vi "Marker Draw and Commands Loop.vi"(4 "Cursor Options":T1={"font"={"Font Name"="Arial", "Size"=15, "Strikeout?"=FALSE, "Italic?"=FALSE, "Underline?"=FALSE, "Outline?"=FALSE, "Shadow?"=FALSE, "Bold?"=FALSE}, "size"=2, "Timestamp"=enum."at BOTTOM", "Vertical Line?"=TRUE, "Horizontal Line?"=TRUE, "alignment(left, top)"={"horizontal"=enum."left", "vertical"=enum."center"}, "TextFormat"=" %3$s\\n %2$.2f", "time format (%H:%M:%S)"="%I:%M:%S %p"} {"size" min=1 max=50}, 6 "Enable Cursors":bool, 9 "Markers":T2[](array[typedef]), 10 "XY Graph":refnum<vi>, 11 "Options":T4={"Color"=16723218, "pen"={"Width"=2, "Style"=enum."Solid"}, "font"={"Font Name"="Arial", "Size"=14, "Strikeout?"=FALSE, "Italic?"=FALSE, "Underline?"=FALSE, "Outline?"=FALSE, "Shadow?"=FALSE, "Bold?"=FALSE, "FontColor"=6908265}, "caption"="Click to set a point marker"}) -> ()   [LabVIEW 2020, in "Graph Extensions.lvlib"]
doc: "This draw loop is the command processor thread and redraw thread to handle the events from the UI. It can be started anywhere with a reference to the graph. Markers work only when the graph palette tool is in cursor mode, as it replaces that mode since Graph extensions have their own improved cursors/markers, that mode is not needed. \n\n<B>Options</B> can be changed by the user using the right click menu with the markers.\n<B>Markers</B> input can be used to initialize a known set of markers (eitehr loaded from disk or programmatically created)\n\n<B>Cursers Enabled</B> activates the other graph extension (cursors) when usual mouse move occurs."
uses:
  Graph Extensions.lvlib
  controls/MarkerOptions.ctl
  controls/MarkerInfo.ctl
  controls/markerType.ctl
  controls/CursorOptions.ctl
  controls/GraphExt-Cmds.ctl
  controls/commands.ctl
  <vilib>/Utility/miscctls.llb/LVPoint32TypeDef.ctl
  controls/cmd_options.ctl
  controls/Simple Global for Marker Options.vi
panel:
  in  "stop":bool
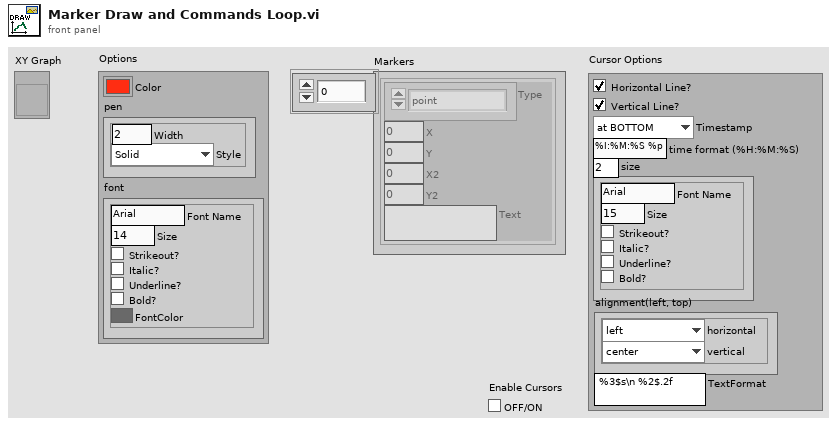
[diagram p1: front panel]
types:
  T1 = typedef "Graph Extensions.lvlib/CursorOptions.ctl" = cluster{"font":cluster{"Font Name":string, "Size":i16, "Strikeout?":bool, "Italic?":bool, "Underline?":bool, "Outline?":bool, "Shadow?":bool, "Bold?":bool}, "size":i16, "Timestamp":enum16{"at TOP", "at BOTTOM", "none"}, "Vertical Line?":bool, "Horizontal Line?":bool, "alignment(left, top)":cluster{"horizontal":enum16{"left", "center", "right"}, "vertical":enum16{"top", "center", "bottom"}}, "TextFormat":string, "time format (%H:%M:%S)":string}
  T2 = typedef "Graph Extensions.lvlib/MarkerInfo.ctl" = cluster{"Type":T3, "X":dbl, "Y":dbl, "X2":dbl, "Y2":dbl, "Text":string}
  T3 = typedef "Graph Extensions.lvlib/markerType.ctl" = enum16{"point", "arrow", "horiz", "vert", "vert range", "horiz range", "box"}
  T4 = typedef "Graph Extensions.lvlib/MarkerOptions.ctl" = cluster{"Color":u32, "pen":cluster{"Width":u16, "Style":enum32{"Solid", "Dash", "Dot", "DashDot", "DashDotDot"}}, "font":cluster{"Font Name":string, "Size":i16, "Strikeout?":bool, "Italic?":bool, "Underline?":bool, "Outline?":bool, "Shadow?":bool, "Bold?":bool, "FontColor":u32}, "caption":string}
  T5 = typedef "Graph Extensions.lvlib/commands.ctl" = enum16{"up", "options", "click", "move", "type", "redraw", "edited", "exit", "Mark"}
  T6 = typedef "LVPoint32TypeDef.ctl" = cluster{"Horizontal":i32, "Vertical":i32}
  T7 = cluster{"cmd":T5, "Type":T3, "Coords":T6, "Active Tool":i32, "mode":enum16{"drag", "none"}}
  T8 = typedef "Graph Extensions.lvlib/GraphExt-Cmds.ctl" = cluster{"cmd":T5, "Type":T3, "Coords":T6, "text":string}
  T9 = typedef "Graph Extensions.lvlib/cmd_options.ctl" = cluster{"Marker Color":u32, "Style":enum32{"Solid", "Dash", "Dot", "DashDot", "DashDotDot"}, "Width":u16, "Size":i16, "Color":u32}
  T10 = typedef "LVRectTypeDef.ctl" = cluster{"Left":i16, "Top":i16, "Right":i16, "Bottom":i16}
  T11 = enum32{"Solid", "Dash", "Dot", "DashDot", "DashDotDot"}
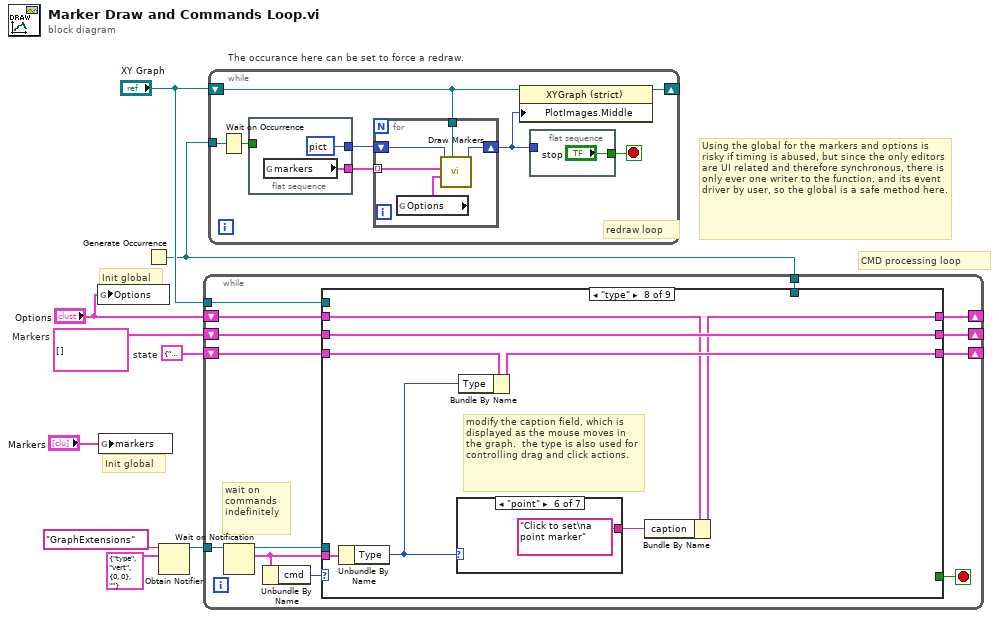
[diagram p0: block diagram]
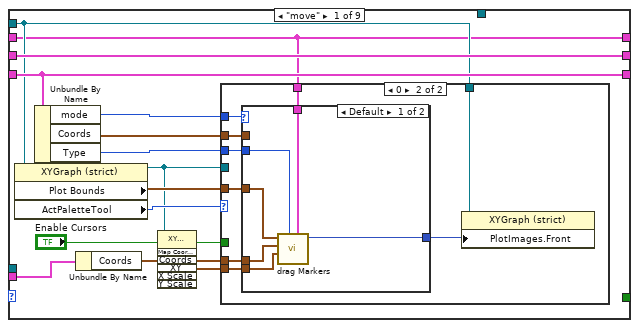
[diagram p2: hidden frame]
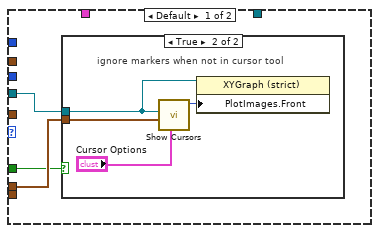
[diagram p3: hidden frame]
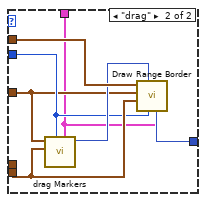
[diagram p5: hidden frame]
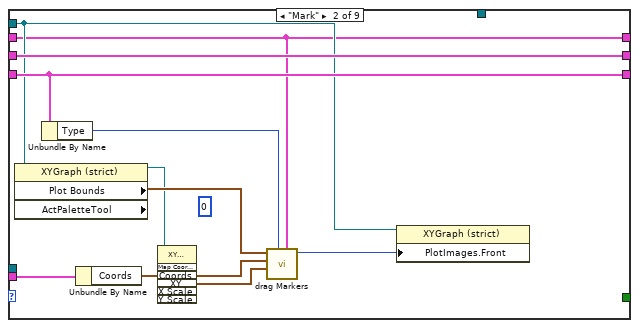
[diagram p6: hidden frame]
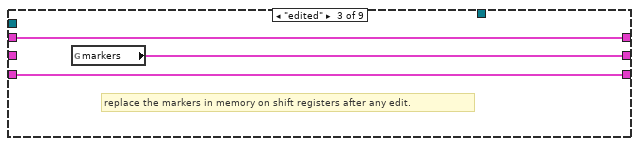
[diagram p7: hidden frame]
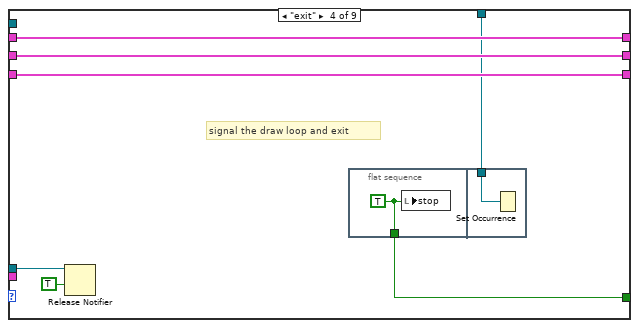
[diagram p8: hidden frame]
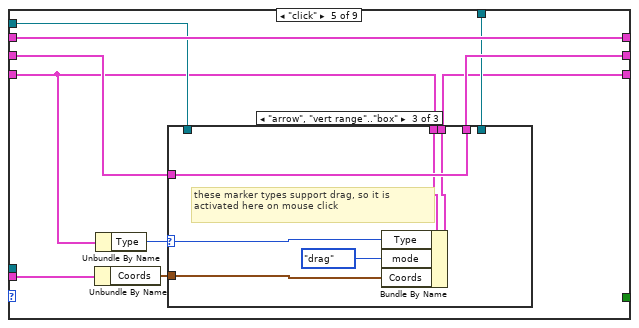
[diagram p9: hidden frame]
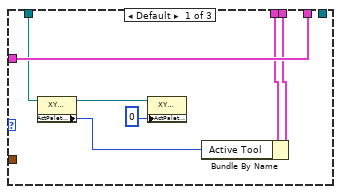
[diagram p10: hidden frame]
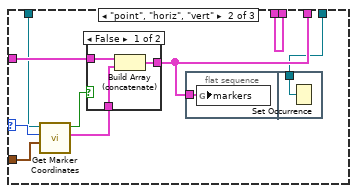
[diagram p11: hidden frame]
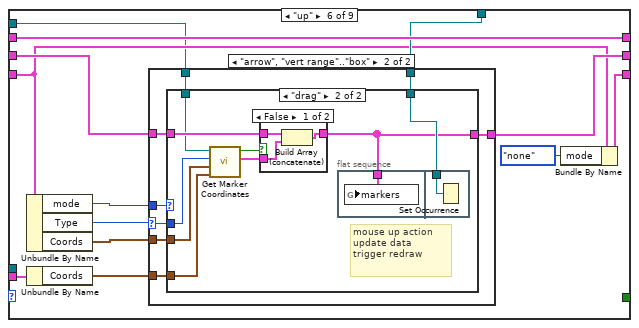
[diagram p13: hidden frame]
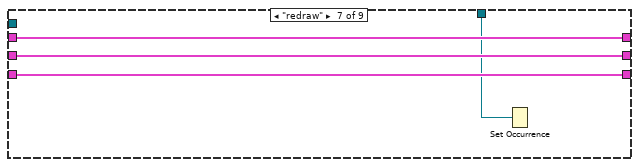
[diagram p17: hidden frame]
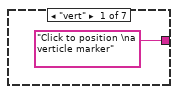
[diagram p18: hidden frame]
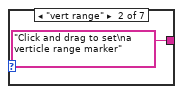
[diagram p19: hidden frame]
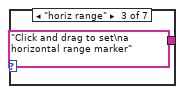
[diagram p20: hidden frame]
diagram:
  w5 = T7 {"cmd"=enum."click", "Type"=enum."point", "Coords"={"Horizontal"=0, "Vertical"=0}, "Active Tool"=0, "mode"=enum."none"}  # state
  w4 = T2[] []  # Markers
  # "Init global"
  # "CMD processing loop"
  # "Using the global for the markers and options is risky if timing is abused, but since the only editors are UI related and therefore synchronous, there is only ever one writer to the function, and its event driver by user, so the global is a safe method here."
  # "Init global"
  # "The occurance here can be set to force a redraw."
  n1 = global write "Simple Global for Marker Options.vi" "Options"("Options") -> ()
  n2 = global write "Simple Global for Marker Options.vi" "markers"("Markers") -> ()
  n3 = Generate Occurrence() -> (w3:refnum<k4>)
  n4 = Obtain Notifier(name (unnamed)="GraphExtensions", notification data type=T8 {"cmd"=enum."type", "Type"=enum."vert", "Coords"={"Horizontal"=0, "Vertical"=0}, "text"=""}) -> (notifier out=w8:refnum<notifier>)  [unwired: 2 in, 2 out]
  n5 = while {
    tunnel: w8 -> [w22]
    shift-right: [w18] -> _
    shift-left: "Options" -> [w19]
    shift-right: [w17] -> _
    shift-left: w4 -> [w16]
    shift-right: [w15] -> _
    shift-left: w5 -> [w14]
    tunnel: w3 -> [w13]
    tunnel: "XY Graph" -> [w12]
    stop <- w11 stop-if-true
    # "wait on\ncommands\nindefinitely"
    n6 = Wait on Notification(notifier=w22) -> (notifier out=w10:refnum<notifier>, notification=w21:T8)  [unwired: 3 in, 2 out]
    n7 = Unbundle By Name(w21) -> ("cmd"=w20:T5)
    n8 = case shown="\"type\"" w20 {
      tunnel: w19 -> [w28 w70 w79 w86 w98 w139 w166 w170 w190]
      tunnel: w21 -> [w36 w76 _ _ w97 w138 _ w175 w195]
      tunnel: [w28 w70 w79 w86 w98 w139 w166 w169 w185] -> w18
      tunnel: [w35 w75 w77 w85 w96 w132 w168 w176 w197] -> w17
      tunnel: w16 -> [w35 w75 _ w85 w92 w133 w168 w176 w197]
      tunnel: [w34 w74 w78 w84 w93 w129 w167 w173 w196] -> w15
      tunnel: w14 -> [w34 w74 w78 w84 w91 w130 w167 w174 w196]
      tunnel: w13 -> [_ _ _ w82 w95 w131 w165 _ w184]
      tunnel: w12 -> [w30 w72 _ _ w94 w127 _ _ _]
      tunnel: [_ _ _ w83 _ _ _ _ _] -> w11
      tunnel: w10 -> [_ _ _ w81 _ _ _ _ _]
      frame "move" {
        n9 = property on="Property Node" class="XYGraph (strict)"(reference=w30) -> (reference out=w25:refnum<vi>, "Plot Bounds"=w29:T10, "ActPaletteTool"=w27:i32)  [unwired: 1 in, 1 out]
        n10 = Unbundle By Name(w34) -> ("mode"=w32:enum16{"drag", "none"}, "Coords"=w33:T6, "Type"=w31:T3)
        n11 = Unbundle By Name(w36) -> ("Coords"=w24:T6)
        n12 = invoke class="XYGraph (strict)" method="Map Coords To XY"(reference=w25, "Coords"=w24) -> ("XY"=w23:cluster{"X":dbl, "Y":dbl})  [unwired: 5 in, 6 out]
        n13 = case shown="0" w27 {
          tunnel: w33 -> [_ w52]
          tunnel: w32 -> [_ w50]
          tunnel: w31 -> [_ w49]
          tunnel: w24 -> [w38 w48]
          tunnel: w30 -> [_ w47]
          tunnel: w29 -> [_ w46]
          tunnel: w28 -> [_ w45]
          tunnel: w25 -> [w39 _]
          tunnel: "Enable Cursors" -> [w37 _]
          tunnel: w23 -> [_ w44]
          frame Default {
            n14 = case shown="True" w37 {
              tunnel: w39 -> [_ w41]
              tunnel: w38 -> [_ w40]
              frame False {
              }
              frame True {
                # "ignore markers when not in cursor tool"
                n15 = call "Show Cursors.vi"("Cursor Options"="Cursor Options", "Coords"=w40, "XY Graph"=w41) -> ("output picture"=w43:picture)  [unwired: 7 in, 1 out]
                n16 = property on="Property Node" class="XYGraph (strict)"(reference=w41, "PlotImages.Front"=w43) -> ()  [unwired: 1 in, 2 out]
              }
            }
          }
          frame 0 {
            n17 = case shown="Default" w50 {
              tunnel: w52 -> [_ w65]
              tunnel: [w58 w64] -> w51
              tunnel: w45 -> [w57 w59]
              tunnel: w49 -> [w56 w61]
              tunnel: w48 -> [w55 w62]
              tunnel: w46 -> [w54 w60]
              tunnel: w44 -> [w53 _]
              frame Default {
                n18 = call "drag Markers.vi"("Marker Options"=w57, "Type"=w56, "XY"=w53, "Coords"=w55, "Plot Area Bounds"=w54) -> ("new picture"=w58:picture)  [unwired: 6 in]
              }
              frame "drag" {
                n19 = call "drag Markers.vi"("Marker Options"=w59, "Type"=w61, "Coords"=w62, "Plot Area Bounds"=w60) -> ("new picture"=w63:picture)  [unwired: 7 in]
                n20 = call "Draw Range Border.vi"("Marker Options"=w59, "Type"=w61, "picture"=w63, "end Coords"=w62, "Plot Bounds"=w60, "Start Coords"=w65) -> ("new picture"=w64:picture)  [unwired: 5 in]
              }
            }
            n21 = property on="Property Node" class="XYGraph (strict)"(reference=w47, "PlotImages.Front"=w51) -> ()  [unwired: 1 in, 2 out]
          }
        }
      }
      frame "Mark" {
        (unwired) 0 ("ActPaletteTool")
        n22 = property on="Property Node" class="XYGraph (strict)" props=["Plot Bounds", "ActPaletteTool"](reference=w72) -> (reference out=w69:refnum<vi>, "Plot Bounds"=w71:T10)  [unwired: 1 in, 2 out]
        n23 = Unbundle By Name(w74) -> ("Type"=w73:T3)
        n24 = Unbundle By Name(w76) -> ("Coords"=w68:T6)
        n25 = invoke class="XYGraph (strict)" method="Map Coords To XY"(reference=w69, "Coords"=w68) -> ("XY"=w67:cluster{"X":dbl, "Y":dbl})  [unwired: 5 in, 6 out]
        n26 = call "drag Markers.vi"("Marker Options"=w70, "Type"=w73, "XY"=w67, "Coords"=w68, "Plot Area Bounds"=w71) -> ("new picture"=w66:picture)  [unwired: 6 in]
        n27 = property on="Property Node" class="XYGraph (strict)"(reference=w72, "PlotImages.Front"=w66) -> ()  [unwired: 1 in, 2 out]
      }
      frame "edited" {
        # "replace the markers in memory on shift registers after any edit."
        n28 = global read "Simple Global for Marker Options.vi" "markers"() -> (w77:T2[])
      }
      frame "exit" {
        # "signal the draw loop and exit"
        n29 = Release Notifier(notifier=w81, force destroy? (F)=TRUE) -> ()  [unwired: 1 in, 3 out]
        n30 = flat-sequence {
          tunnel: [w87] -> w83
          tunnel: w82 -> [w88]
          frame #0 {
            w87 = TRUE
            n31 = local write "stop"(w87) -> ()
          }
          frame #1 {
            n32 = Set Occurrence(w88) -> ()
          }
        }
      }
      frame "click" {
        n33 = Unbundle By Name(w97) -> ("Coords"=w89:T6)
        n34 = Unbundle By Name(w91) -> ("Type"=w90:T3)
        n35 = case shown="\"arrow\", \"vert range\"..\"box\"" w90 {
          selector: w90 -> [_ w111 w122]
          tunnel: w92 -> [w105 w114 w126]
          tunnel: [w105 w113 w126] -> w96
          tunnel: w95 -> [_ w110 _]
          tunnel: w94 -> [w104 w109 _]
          tunnel: w91 -> [w103 w112 w125]
          tunnel: [w102 w112 w124] -> w93
          tunnel: w89 -> [_ w108 w121]
          frame Default {
            n36 = property class="XYGraph (strict)"(reference=w104) -> (reference out=w100:refnum<vi>, "ActPaletteTool"=w101:i32)  [unwired: 1 in, 1 out]
            n37 = property class="XYGraph (strict)"(reference=w100, "ActPaletteTool"=0 ("Palette:Active Tool")) -> ()  [unwired: 1 in, 2 out]
            n38 = Bundle By Name(cluster=w103, "Active Tool"=w101) -> (w102:T7)
          }
          frame "point", "horiz", "vert" {
            n39 = call "Get Marker Coordinates.vi"("Coords"=w108, "Type"=w111, "XYGraph in"=w109) -> ("Markers"=w106:T2, "Cancelled"=w107:bool)  [unwired: 7 in]
            n40 = case shown="False" w107 {
              tunnel: w114 -> [w117 w118]
              tunnel: w106 -> [w116 _]
              tunnel: [w115 w118] -> w113
              frame False {
                n41 = Build Array (concatenate)(w117, w116) -> (w115:T2[])
              }
              frame True {
              }
            }
            n42 = flat-sequence {
              tunnel: w113 -> [w119]
              tunnel: w110 -> [w120]
              frame #0 {
                n43 = global write "Simple Global for Marker Options.vi" "markers"(w119) -> ()
              }
              frame #1 {
                n44 = Set Occurrence(w120) -> ()
              }
            }
          }
          frame "arrow", "vert range".."box" {
            # "these marker types support drag, so it is\nactivated here on mouse click"
            n45 = Bundle By Name(cluster=w125, "Type"=w122, "mode"=enum16{"drag", "none"}."drag", "Coords"=w121) -> (w124:T7)
          }
        }
      }
      frame "up" {
        n46 = Unbundle By Name(w130) -> ("mode"=w134:enum16{"drag", "none"}, "Type"=w137:T3, "Coords"=w136:T6)
        n47 = Unbundle By Name(w138) -> ("Coords"=w135:T6)
        n48 = case shown="\"arrow\", \"vert range\"..\"box\"" w137 {
          selector: w137 -> [_ w147]
          tunnel: w136 -> [_ w143]
          tunnel: w135 -> [_ w144]
          tunnel: w134 -> [_ w148]
          tunnel: w133 -> [w140 w146]
          tunnel: [w140 w145] -> w132
          tunnel: w131 -> [_ w142]
          tunnel: w127 -> [_ w141]
          frame Default {
            # "mouse up is not supported for these marker types\nor is not needed, since they are single click"
          }
          frame "arrow", "vert range".."box" {
            n49 = case shown="\"drag\"" w148 {
              tunnel: w147 -> [_ w155]
              tunnel: w146 -> [w149 w158]
              tunnel: [w149 w156] -> w145
              tunnel: w144 -> [_ w150]
              tunnel: w143 -> [_ w154]
              tunnel: w142 -> [_ w157]
              tunnel: w141 -> [_ w153]
              frame Default {
                # "if drag mode was not already active\nthen the up event can be ignored."
              }
              frame "drag" {
                # "mouse up action\nupdate data\ntrigger redraw"
                n50 = call "Get Marker Coordinates.vi"("Coords 2"=w150, "Coords"=w154, "Type"=w155, "XYGraph in"=w153) -> ("Markers"=w151:T2, "Cancelled"=w152:bool)  [unwired: 6 in]
                n51 = case shown="False" w152 {
                  tunnel: w158 -> [w161 w162]
                  tunnel: [w160 w162] -> w156
                  tunnel: w151 -> [w159 _]
                  frame False {
                    n52 = Build Array (concatenate)(w161, w159) -> (w160:T2[])
                  }
                  frame True {
                  }
                }
                n53 = flat-sequence {
                  tunnel: w156 -> [w163]
                  tunnel: w157 -> [w164]
                  frame #0 {
                    n54 = global write "Simple Global for Marker Options.vi" "markers"(w163) -> ()
                  }
                  frame #1 {
                    n55 = Set Occurrence(w164) -> ()
                  }
                }
              }
            }
          }
        }
        n56 = Bundle By Name(cluster=w130, "mode"=enum16{"drag", "none"}."none") -> (w129:T7)
      }
      frame "redraw" {
        n57 = Set Occurrence(w165) -> ()
      }
      frame "type" {
        # "modify the caption field, which is displayed as the mouse moves in the graph.  the type is also used for controlling drag and click actions."
        n58 = Unbundle By Name(w175) -> ("Type"=w172:T3)
        n59 = case shown="\"point\"" w172 {
          tunnel: ["Click to position \na verticle marker" ("Text") "Click and drag to set\na verticle range marker" ("Text") "Click and drag to set\na horizontal range marker" ("Text") "Click and drag to set\na box marker" ("Text") "Click and drag to draw an arrow" ("Text") "Click to set\na point marker" ("Text") "Click to position \na horizontal marker" ("Text")] -> w171
          frame "vert" {
          }
          frame "vert range" {
          }
          frame "horiz range" {
          }
          frame "box" {
          }
          frame "arrow" {
          }
          frame "point" {
          }
          frame "horiz" {
          }
        }
        n60 = Bundle By Name(cluster=w174, "Type"=w172) -> (w173:T7)
        n61 = Bundle By Name(cluster=w170, "caption"=w171) -> (w169:T4)
      }
      frame "options" {
        # "updates the options for drawing"
        # "Only writer to this global data"
        n62 = Unbundle By Name(w195) -> ("text"=w194:string)
        n63 = Unflatten From String(type=T9 {"Marker Color"=0, "Style"=enum."Solid", "Width"=0, "Size"=0, "Color"=0} ("cluster"), binary string=w194) -> (value=w193:T9)  [unwired: 3 in, 2 out]
        n64 = Unbundle By Name(w193) -> ("Marker Color"=w191:u32, "Style"=w189:T11, "Width"=w188:u16, "Size"=w187:i16, "Color"=w186:u32)
        n65 = Bundle By Name(cluster=w190, "Color"=w191, "pen.Style"=w189, "pen.Width"=w188, "font.Size"=w187, "font.FontColor"=w186) -> (w185:T4)
        n66 = flat-sequence {
          tunnel: w185 -> [w198]
          tunnel: w184 -> [w199]
          frame #0 {
            n67 = global write "Simple Global for Marker Options.vi" "Options"(w198) -> ()
          }
          frame #1 {
            n68 = Set Occurrence(w199) -> ()
          }
        }
      }
    }
  }
  n69 = while {
    shift-right: [w202] -> _
    shift-left: "XY Graph" -> [w201]
    tunnel: w3 -> [w207]
    stop <- w203 stop-if-true
    # "redraw loop"
    n70 = Wait on Occurrence(2:w207) -> (0:w204:bool)  [unwired: 2 in]
    n71 = flat-sequence {
      tunnel: [w209] -> w206
      tunnel: [picture data[5B] ("new picture")] -> w205
      tunnel: w204 -> [_]
      frame #0 {
        n72 = global read "Simple Global for Marker Options.vi" "markers"() -> (w209:T2[])
      }
    }
    n73 = for {
      tunnel: w206 -> [w215] mode=indexing
      shift-right: [w213] -> w200
      shift-left: w205 -> [w214]
      tunnel: w201 -> [w212]
      n74 = global read "Simple Global for Marker Options.vi" "Options"() -> (w211:T4)
      n75 = call "Draw Markers.vi"("XYGraph in"=w212, "Marker Options"=w211, "Marker"=w215, "picture"=w214) -> ("new picture"=w213:picture)  [unwired: 7 in]
    }
    n76 = property class="XYGraph (strict)"(reference=w201, "PlotImages.Middle"=w200) -> (reference out=w202:refnum<vi>)  [unwired: 1 in, 1 out]
    n77 = flat-sequence {
      tunnel: ["stop"] -> w203
      tunnel: w200 -> [_]
      frame #0 {
      }
    }
  }
